vi "Configure Level Trigger.vi"(0 "device session in":refnum<class "Device Session.lvclass">, 1 "trigger source":u8, 5 "trigger when":T1, 7 "trigger level (V)":dbl, 11 "error in":errorcluster, 12 "instance":enum16{"A", "B"}(ring)) -> (4 "device session out":refnum<class "Device Session.lvclass">, 15 "error out":errorcluster)   [LabVIEW 2021, in "Device Session.lvclass"]
doc: "Configures the level trigger for a channel. You can specify the trigger slope, the trigger level, and whether the device should trigger on an input below or above the specified trigger level. You must run the <B>Configure Channel</B> VI before running this VI.\n\n<B>Input Parameters</B>\n\n<B>device session in</B> is a reference to the Device Session object, which contains a session to each instrument design library used in this sample project. This parameter is obtained from the 'Open Session' VI.\n\n<B>trigger source</B> specifies the channel to monitor for trigger conditions.\n\n<B>trigger when</B> specifies whether the device should trigger if the input is below or above the specified 'level'.\n\n<B>trigger level (V)</B> specifies the voltage threshold for the trigger.\n\n<B>instance</B> specifies either instance A or B of the trigger to use.\n\n<B>error in</B> describes error conditions that occur before this node runs. This input provides standard 'error in' functionality.\n\n<B>Output Parameters</B>\n\n<B>device session out</B> passes a reference to the session to the next VI.\n\n<B>error out</B> contains error information. This output provides standard 'error out' functionality."
uses:
  Device Session.lvclass
  <instrlib>/_niInstr/Data Trigger/v1/Shared/Public/Level Configuration Trigger When.ctl
  Device Session.lvclass/Device Session.ctl
  <instrlib>/_niInstr/Data Trigger/v1/Shared/Public/Level Configuration FXP(+-,18,1).ctl
  <vilib>/Utility/error.llb/Error Cluster From Error Code.vi
  <vilib>/rvi/errors/niLvFpgaAdjustHostInterfaceError.vi
  <vilib>/rvi/interface/nirviReadWriteControl/nirviReadWriteControl.xnode
  FPGA Refnum.ctl
  <vilib>/rvi/interface/Simulation/niFpgaSimulationCallBeginRW.vi
  <instrlib>/_niInstr/Data Trigger/v1/Shared/niInstr Data Trigger v1 Shared.lvlib
  NiFpgaLv.dll
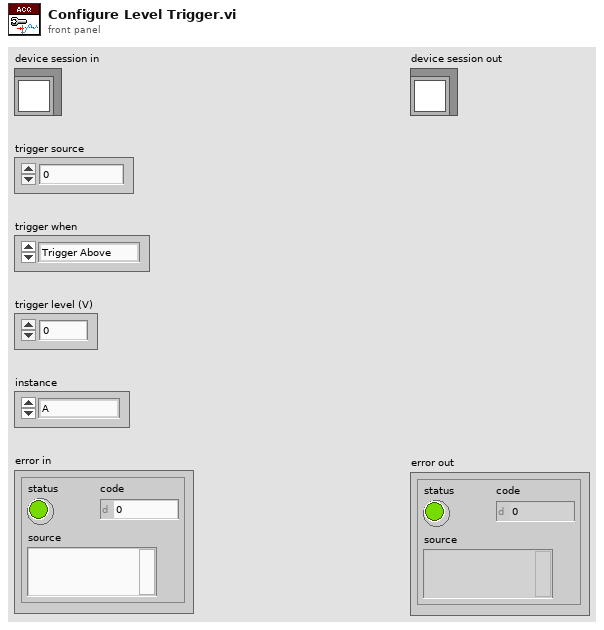
[diagram p1: front panel]
types:
  T1 = typedef "niInstr Data Trigger v1 Shared.lvlib/Level Configuration Trigger When.ctl" = enum8{"Trigger Above", "Trigger Below"}
  T2 = typedef "niInstr Data Trigger v1 Shared.lvlib/Level Configuration FXP(+-,18,1).ctl" = cluster{"level":fxp<+/-,18,5>, "trigger when":T1}
  T3 = enum16{"Immediate", "A", "B", "OR", "AND", "A THEN B", "B THEN A", "High Resolution"}
  T4 = typedef "Device Session.lvclass/Device Session Object.ctl" = cluster{"fpga reference":T5, "reg bus":refnum<class "niInstr FIFO Register Bus v1 Host.lvclass">, "subsystem map":refnum<class "niInstr Subsystem Map v1 Host.lvclass">, "cal data":refnum<class "niHSAI Cal Data v1 Host.lvclass">, "config":refnum<class "niHSAI Group A Config v1 Host.lvclass">, "acquisition 0":refnum<class "niInstr Multirecord Acquisition v1 Host.lvclass">, "acquisition 1":refnum<class "niInstr Multirecord Acquisition v1 Host.lvclass">, "acquisition 2":refnum<class "niInstr Multirecord Acquisition v1 Host.lvclass">, "acquisition 3":refnum<class "niInstr Multirecord Acquisition v1 Host.lvclass">, "acquisition 4":refnum<class "niInstr Multirecord Acquisition v1 Host.lvclass">, "acquisition 5":refnum<class "niInstr Multirecord Acquisition v1 Host.lvclass">, "acquisition 6":refnum<class "niInstr Multirecord Acquisition v1 Host.lvclass">, "acquisition 7":refnum<class "niInstr Multirecord Acquisition v1 Host.lvclass">, "number of selected acq channels":u8, "selected acq channels":bool[], "number of channels":u32, "configured channels":bool[], "acq configuration":cluster{"number of samples":u64, "number of records":u64, "pretrigger samples":u64}, "actual channel configuration":T6[], "sample clock rate (Hz)":dbl, "scaling coefficients":T10[]}
  T5 = typedef "Device Session.lvclass/FPGA Refnum.ctl" = refnum<k20>
  T6 = typedef "niHSAI Types v1 Host.lvlib/Channel Configuration.ctl" = cluster{"channel":u32, "coupling":T7, "impedance":T8, "bandwidth":T9, "vertical range":dbl, "vertical offset":dbl}
  T7 = typedef "niHSAI Types v1 Host.lvlib/Coupling.ctl" = enum8{"Default", "DC", "AC"}
  T8 = typedef "niHSAI Types v1 Host.lvlib/Impedance.ctl" = enum8{"Default", "1 mega ohm", "50 ohm"}
  T9 = typedef "niHSAI Types v1 Host.lvlib/Bandwidth.ctl" = enum8{"Default", "Full Bandwidth", "Anti-alias Filter", "150 MHz"}
  T10 = typedef "niInstr Multirecord Acquisition v1 Host.lvclass/Scaling Coefficient.ctl" = cluster{"gain":dbl, "offset":dbl}
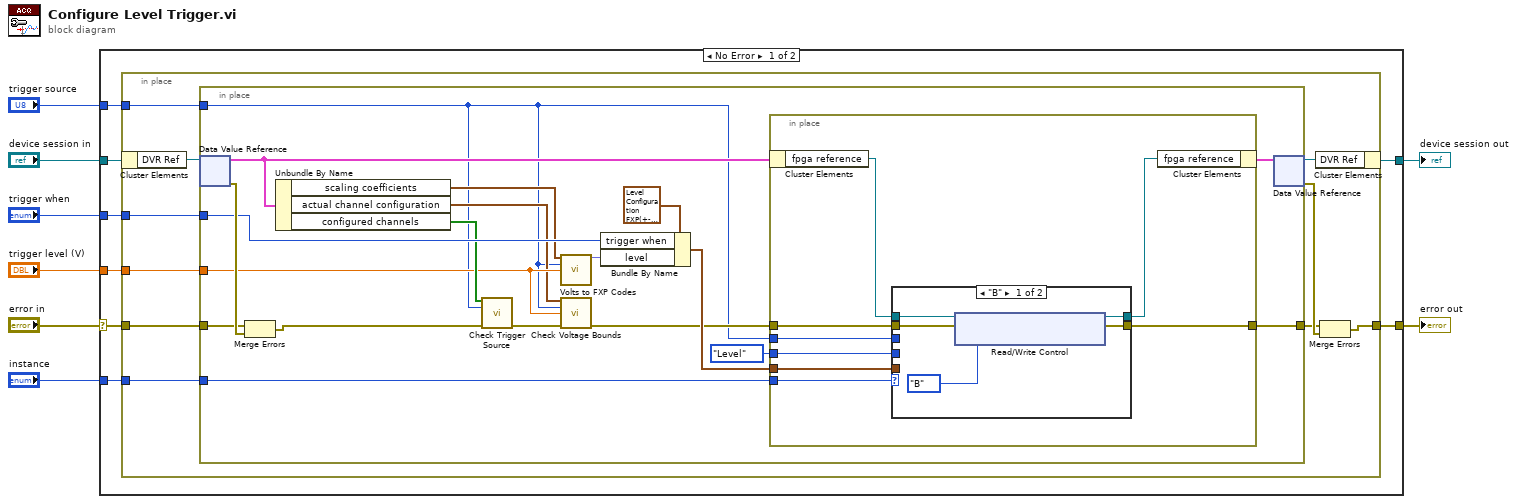
[diagram p0: block diagram]
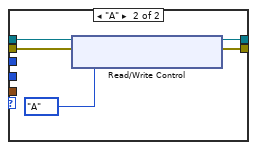
[diagram p2: hidden frame]
diagram:
  n1 = case shown="No Error" "error in" {
    selector: "error in" -> [w16 w65]
    tunnel: "device session in" -> [w10 w64]
    tunnel: [w9 w64] -> w7
    tunnel: [w11 w65] -> w8
    tunnel: "trigger source" -> [w15 _]
    tunnel: "trigger when" -> [w14 _]
    tunnel: "instance" -> [w13 _]
    tunnel: "trigger level (V)" -> [w12 _]
    frame No Error {
      n2 = in-place {
        in-place-border: w16 -> [w26]
        in-place-border: w15 -> [w25]
        in-place-border: w14 -> [w23]
        in-place-border: w13 -> [w22]
        in-place-border: w12 -> [w20]
        in-place-border: [w19] -> w11
        n3 = in-place-cluster #1(w10) -> ("DVR Ref"=w18:refnum<data-value>)
        n4 = in-place {
          in-place-border: w26 -> [w44]
          in-place-border: w25 -> [w27]
          in-place-border: w23 -> [w39]
          in-place-border: w22 -> [w42]
          in-place-border: [w41] -> w21
          in-place-border: w20 -> [w30]
          n5 = in-place-dvr #2(w18) -> (w33:T4, w45:errorcluster)
          n6 = Merge Errors(w44, w45) -> (w31:errorcluster)
          n7 = Unbundle By Name(w33) -> ("scaling coefficients"=w28:T10[], "actual channel configuration"=w29:T6[], "configured channels"=w36:bool[])
          n8 = call "Check Trigger Source.vi"("configured channels"=w36, "trigger source"=w27, "error in"=w31) -> ("error out"=w35:errorcluster)  [unwired: 12 in]
          n9 = call "Volts to FXP Codes.vi"("scaling coefficients"=w28, "channel index"=w27, "level (V)"=w30) -> ("level (fxp)"=w37:fxp<+/-,18,1>)  [unwired: 10 in, 2 out]
          n10 = call "Check Voltage Bounds.vi"("channel configuration"=w29, "trigger source"=w27, "level (V)"=w30, "error in"=w35) -> ("error out"=w34:errorcluster)  [unwired: 11 in]
          n11 = Bundle By Name(cluster=T2 {"level"=0.0, "trigger when"=enum."Trigger Above"} ("configuration"), "trigger when"=w39, "level"=w37) -> (w40:T2)
          n12 = in-place {
            in-place-border: enum16{"Edge", "Level", "Custom"}."Level" ("trigger.select 0") -> [w53]
            in-place-border: w42 -> [w52]
            in-place-border: [w51] -> w41
            in-place-border: w40 -> [w50]
            in-place-border: w34 -> [w49]
            in-place-border: w27 -> [w48]
            n13 = in-place-cluster #3(w33) -> ("fpga reference"=w46:T5)
            n14 = case shown="\"B\"" w52 {
              tunnel: w49 -> [w58 w63]
              tunnel: w48 -> [_ _]
              tunnel: [w57 w62] -> w47
              tunnel: [w56 w61] -> w51
              tunnel: w53 -> [_ _]
              tunnel: w50 -> [_ _]
              tunnel: w46 -> [w54 w59]
              frame "B" {
                n15 = xnode "Read/Write Control"("FPGA VI Reference In"=w54, "error in"=w58, "trigger.combination type"=T3."B" ("trigger.combination.type")) -> ("FPGA VI Reference Out"=w57:T5, "error out"=w56:errorcluster)
              }
              frame "A" {
                n16 = xnode "Read/Write Control"("FPGA VI Reference In"=w59, "error in"=w63, "trigger.combination type"=T3."A" ("trigger.combination.type")) -> ("FPGA VI Reference Out"=w62:T5, "error out"=w61:errorcluster)
              }
            }
            n17 = in-place-cluster #3("fpga reference"=w47) -> (w32:T4)
          }
          n18 = in-place-dvr #2(w32) -> (w17:refnum<data-value>, w24:errorcluster)
        }
        n19 = in-place-cluster #1("DVR Ref"=w17) -> (w9:refnum<class "Device Session.lvclass">)
        n20 = Merge Errors(w21, w24) -> (w19:errorcluster)
      }
    }
    frame Error {
    }
  }
  "error out" <- w8
  "device session out" <- w7
